vi "Build Scenic score.vi"(11 "Array in":i32[](array[numeric])) -> (3 "Secinic score":i32[](array[numeric]))   [LabVIEW 2020]
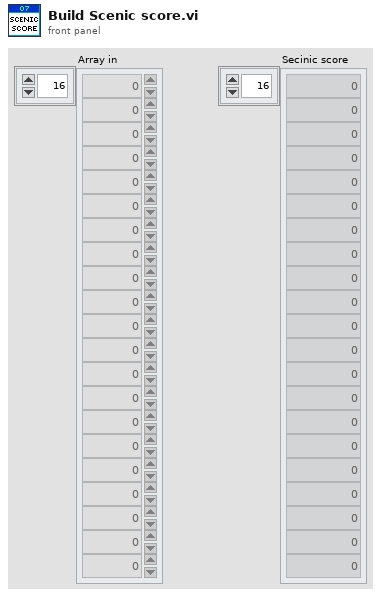
[diagram p1: front panel]
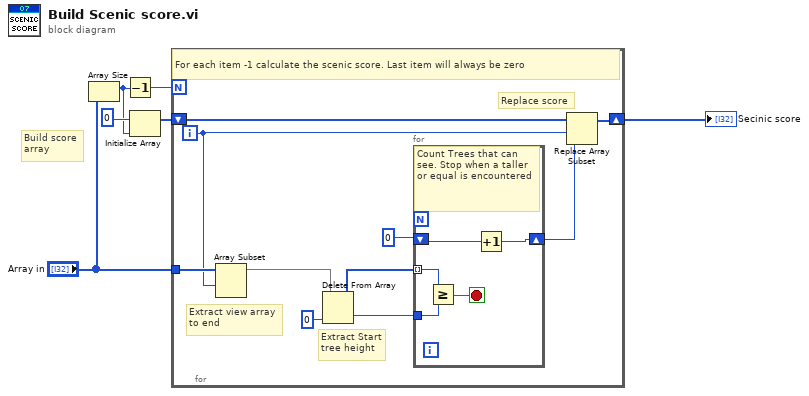
[diagram p0: block diagram]
diagram:
  # "Build score\narray"
  n1 = Array Size(array="Array in") -> (size(s)=w4:i32)
  n2 = Decrement(x=w4) -> (x-1=w2:i32)
  n3 = Initialize Array(0 ("size(s)"), w4) -> (w6:i32[])
  n4 = for {
    N: w2 -> [_]
    tunnel: "Array in" -> [w10]
    shift-right: [w15] -> w1
    shift-left: w6 -> [w16]
    i -> [w9]
    # "Replace score"
    # "Extract Start\ntree height"
    # "Extract view array\nto end"
    # "For each item -1 calculate the scenic score. Last item will always be zero"
    n5 = Array Subset(array=w10, index=w9) -> (w11:i32[])  [unwired: 1 in]
    n6 = Delete From Array(array=w11, index=0) -> (deleted portion=w14:i32, array with subset deleted=w12:i32[])  [unwired: 1 in]
    n7 = for {
      shift-right: [w17] -> w8
      shift-left: 0 -> [w18]
      tunnel: w12 -> [w21] mode=indexing
      tunnel: w14 -> [w20]
      stop <- w19 stop-if-true
      # "Count Trees that can see. Stop when a taller or equal is encountered"
      n8 = Greater Or Equal?(x=w21, y=w20) -> (x >= y?=w19:bool)
      n9 = Increment(x=w18) -> (x+1=w17:i32)
    }
    n10 = Replace Array Subset(array=w16, new element=w8, index=w9) -> (w15:i32[])
  }
  "Secinic score" <- w1
